vi "GT Set Crd Prm.vi"(8 "error in (no error)":errorcluster caption="错误输入（无错误）", 9 "pCrdPrm":T1, 10 "crd":i16, 11 "cardNum":i16) -> (0 "error out":errorcluster caption="错误输出", 3 "function return":i16)   [LabVIEW 2020, in "gts.lvlib"]
doc: "GT_API GT_SetCrdPrm(short cardNum,short crd,TCrdPrm *pCrdPrm);"
uses:
  gts.lvlib
  Controls/CrdPrm.ctl
  dll/32bit/multi_card/gts.dll
  Controls/Controls.lvlib
panel:
  # "关联profile和坐标轴"
  # "用户指定的原点位置"
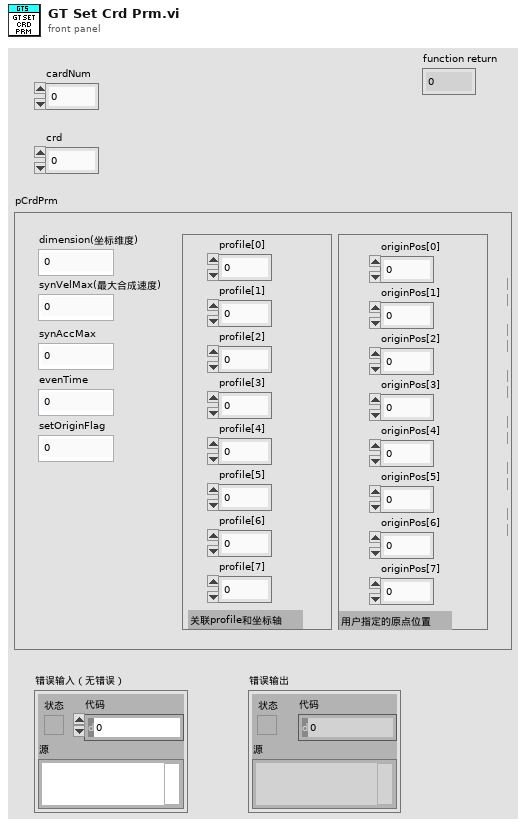
[diagram p1: front panel]
types:
  T1 = typedef "Controls.lvlib/CrdPrm.ctl" = cluster{"dimension(坐标维度)":i16, "profile[0]":i16, "profile[1]":i16, "profile[2]":i16, "profile[3]":i16, "profile[4]":i16, "profile[5]":i16, "profile[6]":i16, "profile[7]":i16, "@dummy control@":i8, "@dummy control@":i8, "@dummy control@":i8, "@dummy control@":i8, "@dummy control@":i8, "@dummy control@":i8, "synVelMax(最大合成速度)":dbl, "synAccMax":dbl, "evenTime":i16, "setOriginFlag":i16, "originPos[0]":i32, "originPos[1]":i32, "originPos[2]":i32, "originPos[3]":i32, "originPos[4]":i32, "originPos[5]":i32, "originPos[6]":i32, "originPos[7]":i32}
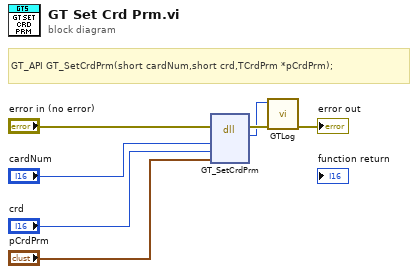
[diagram p0: block diagram]
diagram:
  # "GT_API GT_SetCrdPrm(short cardNum,short crd,TCrdPrm *pCrdPrm);"
  n1 = dll-call lib="C:/1228/dll/32bit/multi_card/gts.dll" fn="GT_SetCrdPrm"(error in="error in (no error)", "cardNum"="cardNum", "crd"="crd", "pCrdPrm"="pCrdPrm") -> (error out=w4:errorcluster, w1:i16)  [unwired: 5 in, 1 out]
  n2 = call "GTLog.vi"("error in (no error)"=w4, "Numeric"=w1) -> ("error out"=→"error out":errorcluster)  [unwired: 9 in]
